vi "Event case-Speed graph cursor moved.vi"(9 "queue in":refnum<queue>, 11 "Cursor in":refnum<vi>) -> (0 "error out":errorcluster)   [LabVIEW 2013]
uses:
  Typedefs/Speed Viewer States enum.ctl
  Globals/gl_Time series viewer globals.vi
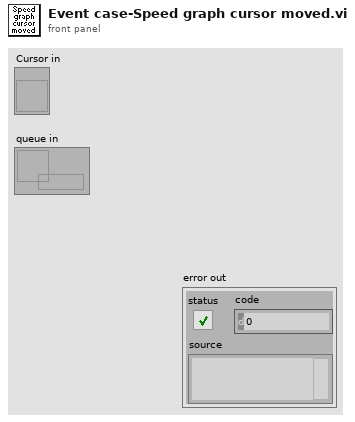
[diagram p1: front panel]
types:
  T1 = typedef "Timelapse viewer refs.ctl" = cluster{"This VI":refnum<vi>, "AVI Mode ind":refnum<vi>, "Play":refnum<vi>, "Stop":refnum<vi>, "Back":refnum<vi>, "Scrollbar":refnum<vi>, "Video length info":refnum<vi>, "Expected speed values":refnum<vi>, "Intensity":refnum<vi>, "Path":refnum<vi>, "Selection sliders":refnum<vi>, "Speed Graph ref":refnum<vi>, "Frame rate set (fps)":refnum<vi>}
  T2 = typedef "Speed Viewer States enum.ctl" = enum16{"Idle", "Initialise", "Playback", "Scroll bar event", "Speed cursor event", "Back to start", "Exit"}
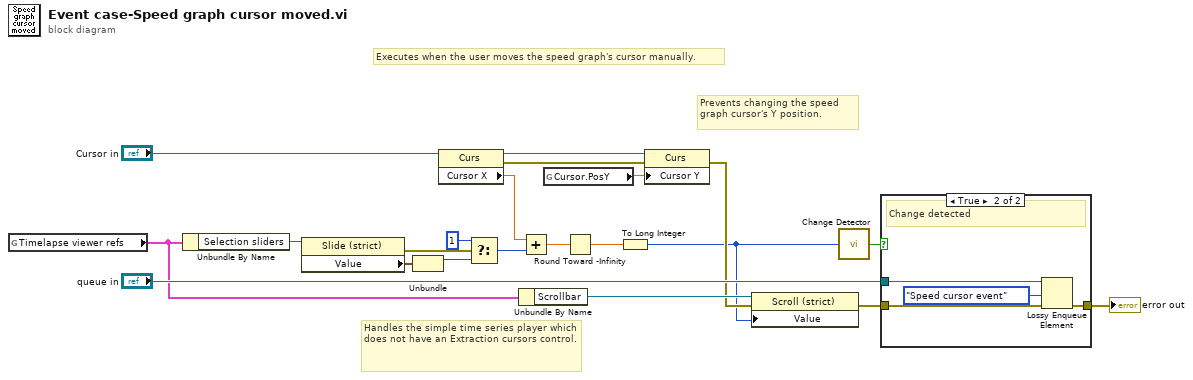
[diagram p0: block diagram]
diagram:
  # "Handles the simple time series player which does not have an Extraction cursors control."
  # "Prevents changing the speed graph cursor's Y position."
  # "Executes when the user moves the speed graph's cursor manually."
  n1 = global read "gl_Time series viewer globals.vi" "Timelapse viewer refs"() -> (w11:T1)
  n2 = Unbundle By Name(w11) -> ("Selection sliders"=w18:refnum<vi>)
  n3 = property on="Property Node" class="Slide (strict)"(reference=w18) -> (error out=w2:errorcluster, "Value"=w19:cluster{i32, i32})  [unwired: 1 in, 1 out]
  n4 = Unbundle(w19) -> (w4:i32)  [unwired: 1 out]
  n5 = property on="Property Node" class="Curs"(reference="Cursor in") -> (reference out=w14:refnum<vi>, error out=w15:errorcluster, "Cursor X"=w16:dbl)  [unwired: 1 in]
  n6 = Select(t=1, s=w2, f=w4) -> (s? t:f=w3:i32)
  n7 = Unbundle By Name(w11) -> ("Scrollbar"=w20:refnum<vi>)
  n8 = Add(x=w16, y=w3) -> (x+y=w17:dbl)
  n9 = global read "gl_Time series viewer globals.vi" "Cursor.PosY"() -> (w9:dbl)
  n10 = Round Toward -Infinity(1:w17) -> (0:w6:dbl)
  n11 = To Long Integer(number=w6) -> (32bit integer=w7:i32)
  n12 = property on="Property Node" class="Curs"(reference=w14, error in=w15, "Cursor Y"=w9) -> (error out=w10:errorcluster)  [unwired: 1 out]
  n13 = property on="Property Node" class="Scroll (strict)"(reference=w20, error in=w10, "Value"=w7) -> (error out=w21:errorcluster)  [unwired: 1 out]
  n14 = call "Change Detector.vi"("Value"=w7) -> ("Changed?"=w8:bool)
  n15 = case shown="True" w8 {
    tunnel: w21 -> [w22 w24]
    tunnel: "queue in" -> [_ w25]
    tunnel: [w22 w23] -> w5
    frame False {
    }
    frame True {
      # "Change detected"
      n16 = Lossy Enqueue Element(queue=w25, element=Speed_Viewer_States_enum."Speed cursor event" ("States"), error in (no error)=w24) -> (error out=w23:errorcluster)  [unwired: 3 out]
    }
  }
  "error out" <- w5
